vi "viewNextMission.vi"(8 "error in (no error)":errorcluster, 11 "MissionQueue in":refnum<class "MissionQueue.lvclass">) -> (0 "error out":errorcluster, 1 "Valid?":bool, 2 "Mission.lvclass":refnum<class "Mission.lvclass">, 3 "MissionQueue out":refnum<class "MissionQueue.lvclass">)   [LabVIEW 2011, in "MissionQueue.lvclass"]
uses:
  MissionQueue.lvclass
  Mission/Mission.lvclass
  MissionQueue.lvclass/MissionQueue.ctl
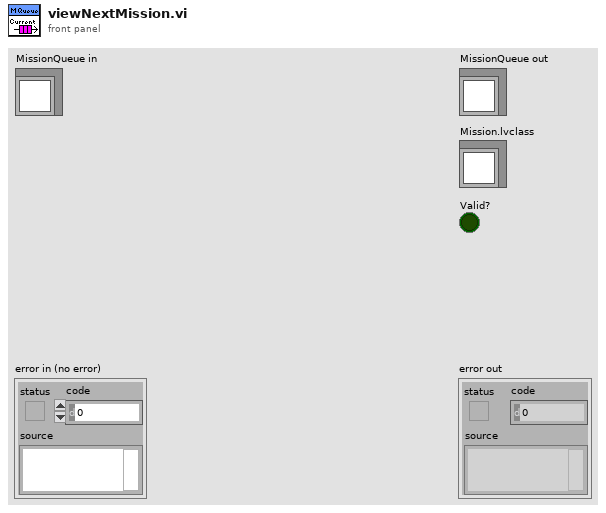
[diagram p1: front panel]
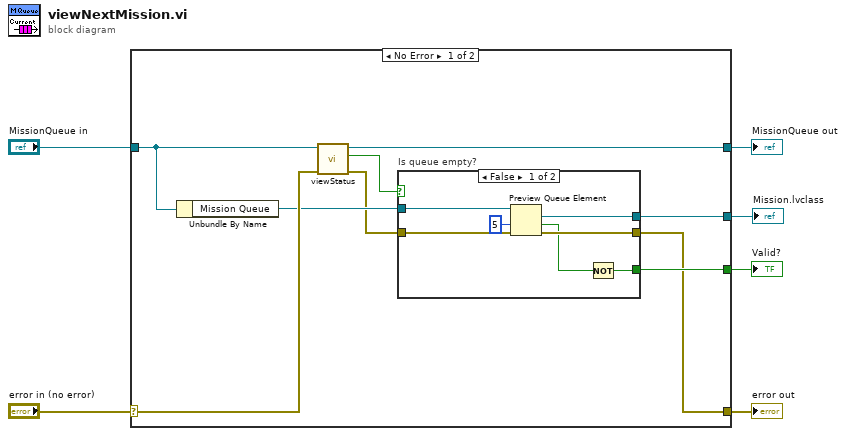
[diagram p0: block diagram]
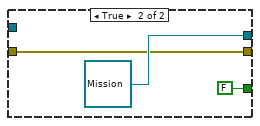
[diagram p2: hidden frame]
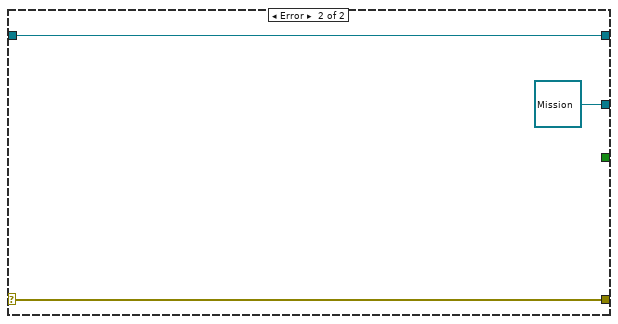
[diagram p3: hidden frame]
diagram:
  n1 = case shown="No Error" "error in (no error)" {
    selector: "error in (no error)" -> [w15 w28]
    tunnel: [w8 w28] -> w5
    tunnel: [w13 w27] -> w3
    tunnel: "MissionQueue in" -> [w12 w27]
    tunnel: [w10 _] -> w2
    tunnel: [w7 refnum<class "Mission.lvclass"> refnum ("Mission.lvclass")] -> w1
    frame No Error {
      n2 = Unbundle By Name(w12) -> ("Mission Queue"=w11:refnum<queue>)
      n3 = call "viewStatus.vi"("error in (no error)"=w15, "MissionQueue in"=w12) -> ("error out"=w9:errorcluster, "Is empty?"=w14:bool, "MissionQueue out"=w13:refnum<class "MissionQueue.lvclass">)  [unwired: 6 in, 1 out]
      n4 = case "Is queue empty?" shown="False" w14 {
        tunnel: w11 -> [w22 _]
        tunnel: [w19 FALSE ("Valid?")] -> w10
        tunnel: w9 -> [w21 w23]
        tunnel: [w20 w23] -> w8
        tunnel: [w16 refnum<class "Mission.lvclass"> refnum ("Mission.lvclass")] -> w7
        frame False {
          n5 = Preview Queue Element(queue=w22, timeout in ms (-1)=5, error in (no error)=w21) -> (element=w16:refnum<class "Mission.lvclass">, timed out?=w18:bool, error out=w20:errorcluster)  [unwired: 1 out]
          n6 = Not(x=w18) -> (.not. x?=w19:bool)
        }
        frame True {
        }
      }
    }
    frame Error {
    }
  }
  "error out" <- w5
  "MissionQueue out" <- w3
  "Valid?" <- w2
  "Mission.lvclass" <- w1
